vi "Conductus Get PID.vi"(3 "Instrument Address":refnum<visa-resource-name>) -> (0 "Stop":bool, 1 "PID Param":dbl[][](array[numeric]) format="%.3f")   [LabVIEW 2025]
doc: "Reads the PID paramters of the Conductus temperature controller. The output is an array consisting P, I, D, and P0. The input is the numeric GPIB address.\nScott Hannahs, NHMFL, November 1996\nAuthor: Scott Hannahs <sth@magnet.fsu.edu>\n\nThis software is licensed for use under the “MIT License\"\nCopyright (c) 2025 Scott Hannahs, sth@sth@magnet.sthnet.net\n\nPermission is hereby granted, free of charge, to any person obtaining a copy of this software and associated documentation files (the \"Software\"), to deal in the Software without restriction, including without limitation the rights to use, copy, modify, merge, publish, distribute, sublicense, and/or sell copies of the Software, and to permit persons to whom the Software is furnished to do so, subject to the following conditions: The above copyright notice and this permission notice shall be included in all copies or substantial portions of the Software.\n\nTHE SOFTWARE IS PROVIDED \"AS IS\", WITHOUT WARRANTY OF ANY KIND, EXPRESS OR IMPLIED, INCLUDING BUT NOT LIMITED TO THE WARRANTIES OF MERCHANTABILITY, FITNESS FOR A PARTICULAR PURPOSE AND NONINFRINGEMENT. IN NO EVENT SHALL THE AUTHORS OR COPYRIGHT HOLDERS BE LIABLE FOR ANY CLAIM, DAMAGES OR OTHER LIABILITY, WHETHER IN AN ACTION OF CONTRACT, TORT OR OTHERWISE, ARISING FROM, OUT OF OR IN CONNECTION WITH THE SOFTWARE OR THE USE OR OTHER DEALINGS IN THE SOFTWARE."
panel:
  # "P"
  # "I"
  # "D"
  # "P0"
  # "Heater"
  # "Analog"
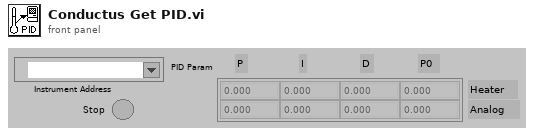
[diagram p1: front panel]
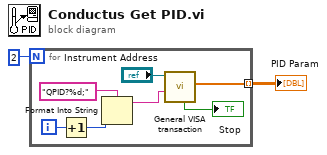
[diagram p0: block diagram]
diagram:
  n1 = for {
    N: 2 -> [_]
    tunnel: [w3] -> w2 mode=indexing
    i -> [w6]
    n2 = Increment(x=w6) -> (x+1=w7:i32)
    n3 = Format Into String(format string="QPID?%d;", w7) -> (resulting string=w4:string)  [unwired: 2 in, 1 out]
    n4 = call "General VISA transaction.vi"("Command String"=w4, "VISA Session"="Instrument Address") -> ("Measurement"=w3:dbl[], "Stop"=→"Stop":bool)  [unwired: 4 in, 4 out]
  }
  "PID Param" <- w2
